vi "configuration UI.vi"() -> ()   [LabVIEW 2015, in "PID Module editor node.lvclass"]
uses:
  PID Module editor node.lvclass
  <vilib>/NI/Configuration Framework/Node/NodeRef.ctl
  <vilib>/NI/Configuration Framework/Node/NISE_CEF_Node.lvclass
  <vilib>/NI/AMC/Message Queue.ctl
  <vilib>/NI/AMC/Message.ctl
  <vilib>/NI/Tools/Keyed Array/KeyedArray.ctl
  <vilib>/NI/Configuration Framework/Node/UserEventRef.ctl
  <vilib>/NI/Configuration Framework/Controls/EventCluster.ctl
  <vilib>/NI/Configuration Framework/Node/StopEvent.ctl
  <vilib>/NI/Configuration Framework/Node/RefreshUIEvent.ctl
  <vilib>/NI/Configuration Framework/Node/CacheState.ctl
  <vilib>/NI/Configuration Framework/Node/NodeChangeEvent.ctl
  Program Files (x86)/National Instruments/LabVIEW 2013/vi.lib/NI/DCAF UI Toolkit/Controls/Configure.ctl
  <vilib>/NI/DCAF UI Toolkit/Controls/Remove.ctl
  <vilib>/NI/DCAF UI Toolkit/Controls/Add.ctl
  PID array element.ctl
  PID Module editor node.lvclass/PID Module editor node.ctl
  <vilib>/NI/Tag Bus Data Framework/Configuration Editor/Classes/Module editor node/module editor node.lvclass
  <vilib>/NI/Tag Bus Data Framework/Configuration Editor/Classes/Engine Parent/Engine Parent Editor Node.lvclass
  <vilib>/NI/Tools/Keyed Array/Tools_KeyedArray.lvlib
  <vilib>/NI/AMC/AMC.lvlib
  <vilib>/NI/Configuration Framework/NISE_CEF_TreeControl.lvlib
  module/configuration/PID Module configuration.lvclass
  <vilib>/NI/DCAF UI Toolkit/Controls/DCAF UI Elements.lvlib
panel:
  in  "node change":T1
  in  "cache state":T2
  in  "refresh UI":T3
  in  "stop event":T4
  in  "Tab Control":enum32{"Static Configuration"}(tab)
  in  "Down Button":bool
  in  "Up Button":bool
  in  "Last Button":bool
  in  "First Button":bool
  in  "Page Up Button":bool
  in  "Page Down Button":bool
  in  "Add Button":T5
  in  "Delete Button":T6
  in  "Settings Button":T7
  in  "hidden_remove":bool
  in  "hidden_settings":bool
  in  "hidden_Add":bool
  in  "PID Array":T8[](array[typedef])
  in  "user event":T9
  in  "main queue":T10
  in  "node ref":T11
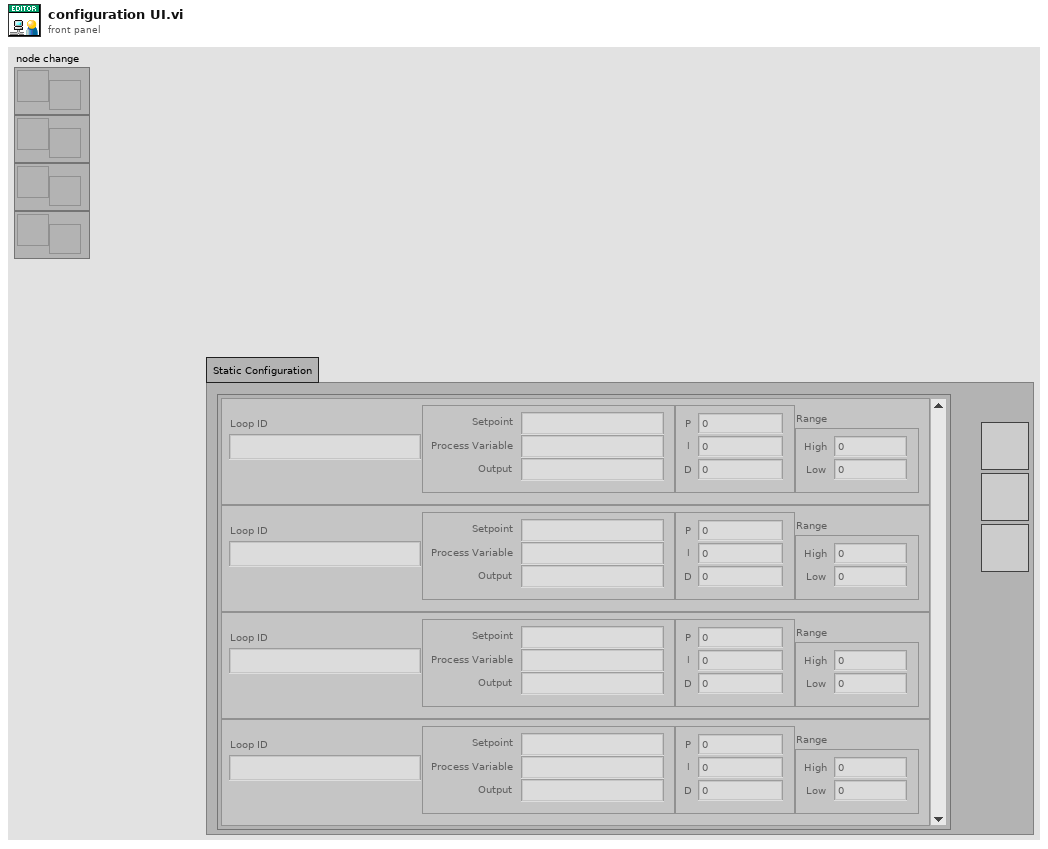
[diagram p1: front panel]
types:
  T1 = typedef "NISE_CEF_Node.lvclass/NodeChangeEvent.ctl" = refnum<user-event>
  T2 = typedef "NISE_CEF_Node.lvclass/CacheState.ctl" = refnum<user-event>
  T3 = typedef "NISE_CEF_Node.lvclass/RefreshUIEvent.ctl" = refnum<user-event>
  T4 = typedef "NISE_CEF_Node.lvclass/StopEvent.ctl" = refnum<user-event>
  T5 = typedef "DCAF UI Elements.lvlib/Add.ctl" = bool
  T6 = typedef "DCAF UI Elements.lvlib/Remove.ctl" = bool
  T7 = typedef "DCAF UI Elements.lvlib/Configure.ctl" = bool
  T8 = typedef "PID Module configuration.lvclass/PID array element.ctl" = cluster{"Loop ID":string, "Tags":cluster{"Setpoint":string, "Process Variable":string, "Output":string}, "Gains":cluster{"P":dbl, "I":dbl, "D":dbl}, "Range":cluster{"High":dbl, "Low":dbl}}
  T9 = typedef "NISE_CEF_Node.lvclass/UserEventRef.ctl" = refnum<user-event>
  T10 = typedef "AMC.lvlib/Message Queue.ctl" = refnum<queue>
  T11 = typedef "NISE_CEF_Node.lvclass/NodeRef.ctl" = refnum<data-value>
  T12 = enum8{"Enabled", "Disabled", "Disabled and Grayed Out"}
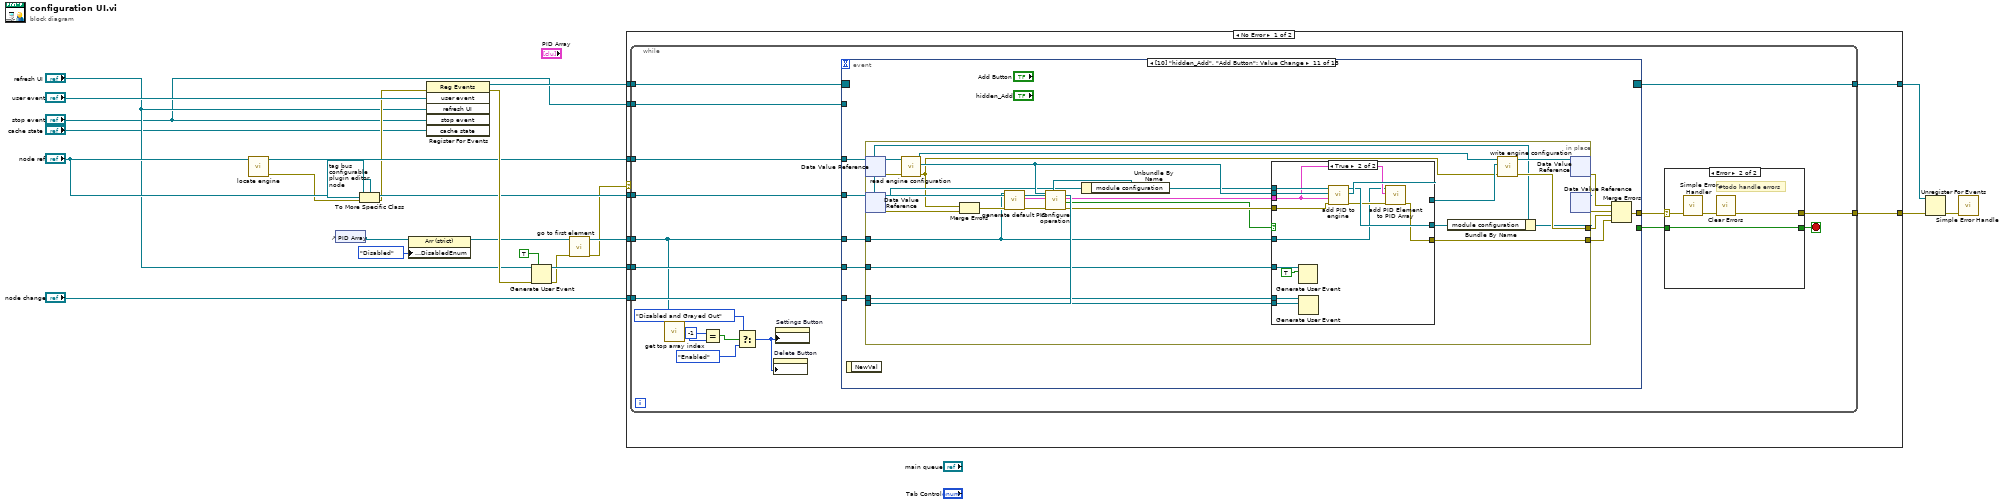
[diagram p0: block diagram]
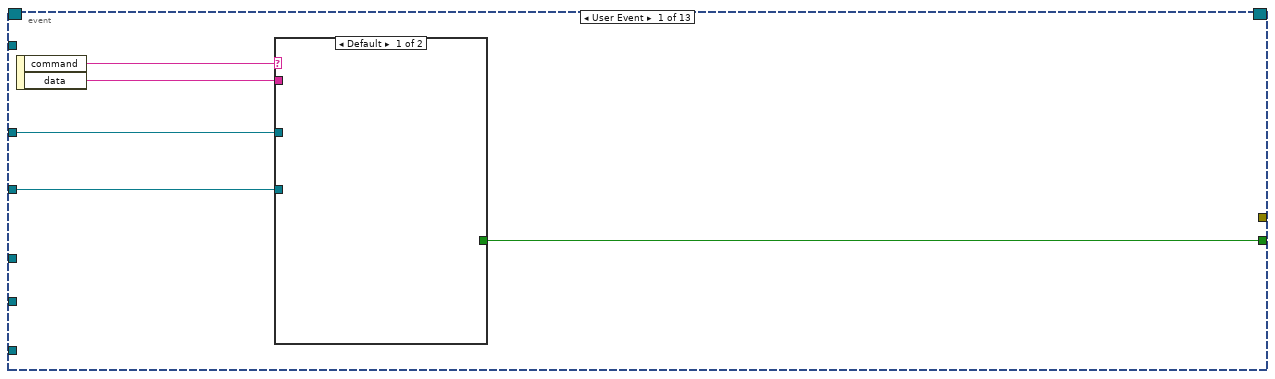
[diagram p2: hidden frame]
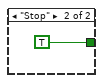
[diagram p3: hidden frame]
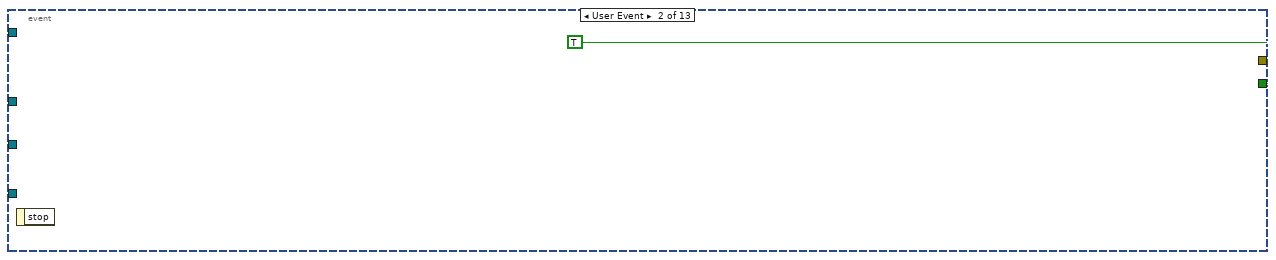
[diagram p4: hidden frame]
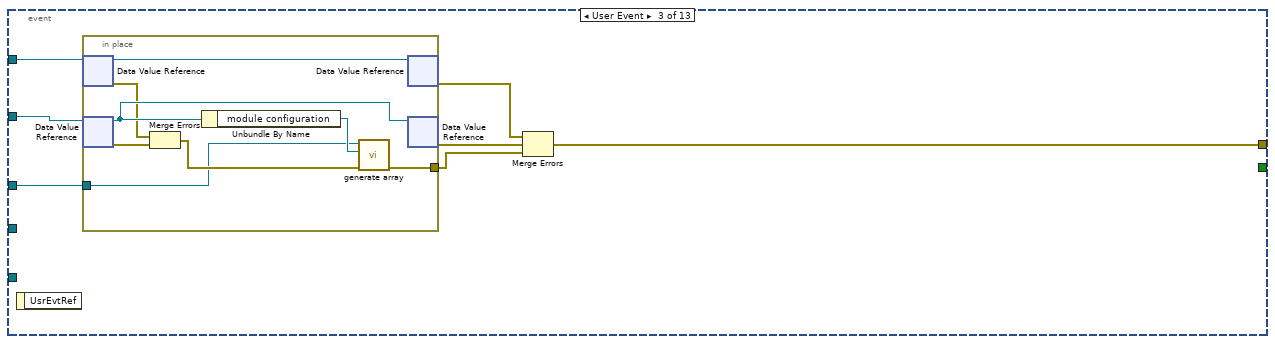
[diagram p5: hidden frame]
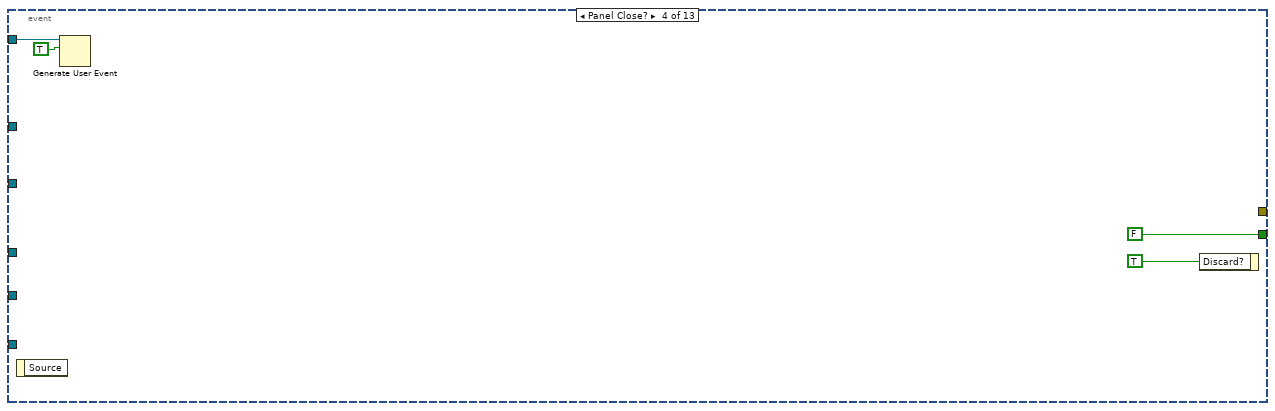
[diagram p6: hidden frame]
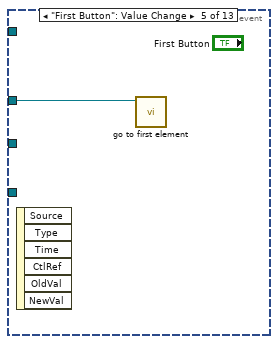
[diagram p7: hidden frame]
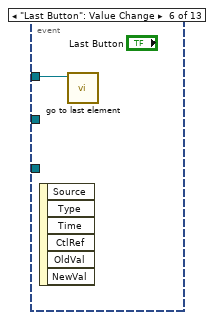
[diagram p8: hidden frame]
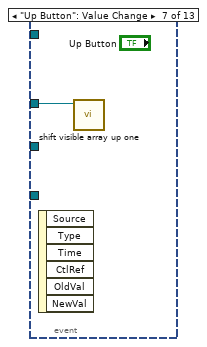
[diagram p9: hidden frame]
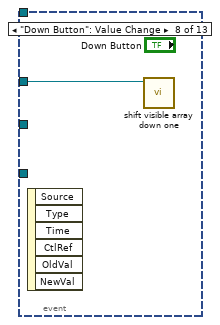
[diagram p10: hidden frame]
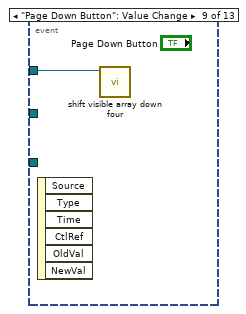
[diagram p11: hidden frame]
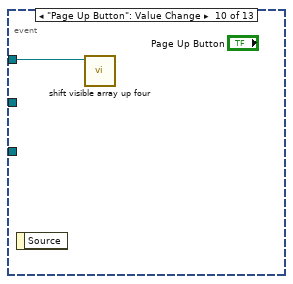
[diagram p12: hidden frame]
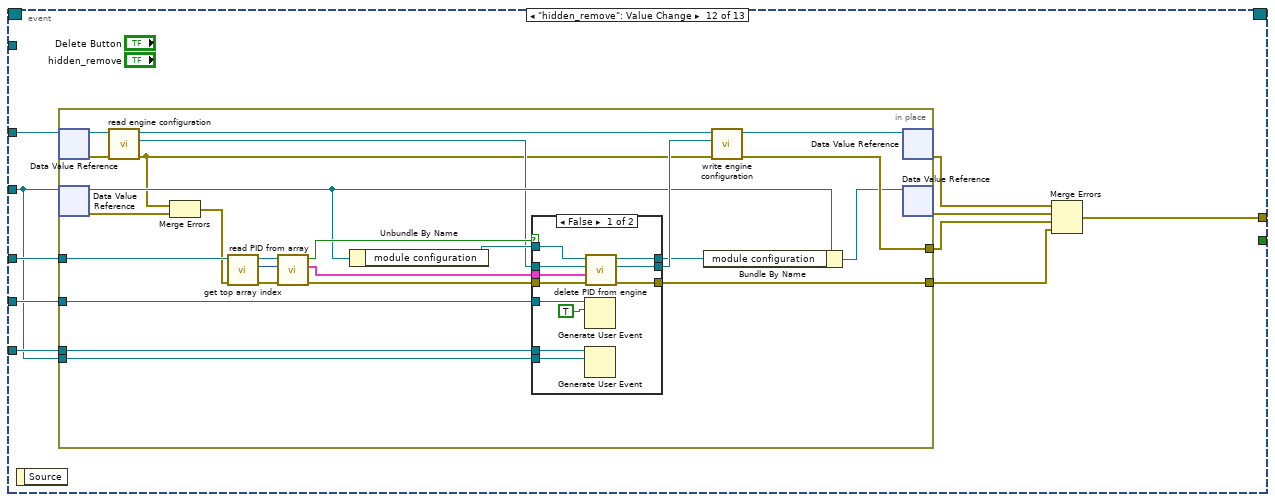
[diagram p14: hidden frame]
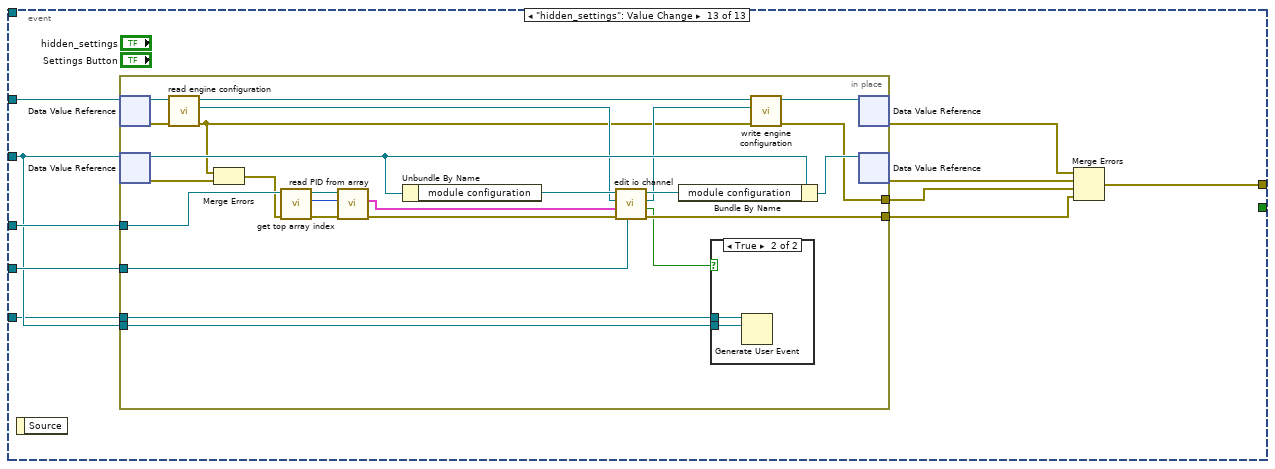
[diagram p16: hidden frame]
diagram:
  n1 = call <vilib>:"locate engine.vi"("component"="node ref") -> ("error out"=w13:errorcluster, "engine"=w19:refnum<data-value>)  [unwired: 9 in]
  n2 = control-ref of="PID Array"() -> (w1:refnum<vi>)
  n3 = To More Specific Class(target class=refnum<data-value> refnum ("data value reference"), reference="node ref", error in=w13) -> (specific class reference=w16:refnum<data-value>, error out=w15:errorcluster)
  n4 = property class="Arr (strict)"(reference=w1, "Array Element.DisabledEnum"=T12."Disabled" ("Disabled")) -> (reference out=w2:refnum<vi>)  [unwired: 1 in, 1 out]
  n5 = register-events(error in=w15, "user event", "refresh UI", "stop event", "cache state") -> (reference out=w24:refnum<event-registration>, error out=w20:errorcluster)  [unwired: 1 in]
  n6 = Generate User Event(user event="refresh UI", event data cluster=TRUE ("event data"), error in=w20) -> (user event out=w12:T3, error out=w5:errorcluster)  [unwired: 1 in]
  n7 = call "go to first element.vi"("error in (no error)"=w5, "Array in"=w2) -> ("error out"=w4:errorcluster, "Array out"=w6:refnum<vi>)  [unwired: 8 in]
  n8 = case shown="No Error" w4 {
    selector: w4 -> [_ w227]
    tunnel: w24 -> [w33 w226]
    tunnel: [w32 w226] -> w23
    tunnel: [w31 w227] -> w22
    tunnel: w19 -> [w30 _]
    tunnel: w6 -> [w29 _]
    tunnel: w16 -> [w28 _]
    tunnel: w12 -> [w27 _]
    tunnel: "node change" -> [w26 _]
    tunnel: "stop event" -> [w25 _]
    frame No Error {
      n9 = while {
        tunnel: w33 -> [w51]
        tunnel: [w50] -> w32
        tunnel: w28 -> [w47]
        tunnel: w30 -> [w46]
        tunnel: w27 -> [w45]
        tunnel: w29 -> [w37]
        tunnel: w26 -> [w44]
        tunnel: [w48] -> w31
        tunnel: w25 -> [w43]
        stop <- w49 stop-if-true
        n10 = call "get top array index.vi"("Array in"=w37) -> ("last value index"=w36:u32)  [unwired: 7 in, 3 out]
        n11 = Equal?(x=-1, y=w36) -> (x = y?=w34:bool)
        n12 = Select(t=T12."Disabled and Grayed Out", s=w34, f=T12."Enabled" ("Disabled")) -> (s? t:f=w38:T12)
        n13 = property on="Delete Button" class="Bool"("DisabledEnum"=w38) -> ()  [unwired: 2 in, 2 out]
        n14 = property on="Settings Button" class="Bool"("DisabledEnum"=w38) -> ()  [unwired: 2 in, 2 out]
        n15 = event shown="[10] \"hidden_Add\", \"Add Button\": Value Change" {
          selector: w51 -> [_ _ _ _ _ _ _ _ _ _ _ _ _]
          dyn-events: [_ _ _ _ _ _ _ _ _ _ _ _ _] -> w50
          timeout: _ -> [_ _ _ _ _ _ _ _ _ _ _ _ _]
          tunnel: [w56 TRUE _ FALSE _ _ _ _ _ _ _ _ _] -> w42
          tunnel: [_ _ w63 _ _ _ _ _ _ _ w84 w140 w190] -> w41
          tunnel: w47 -> [w54 _ w65 _ _ _ _ _ _ _ w90 w138 w188]
          tunnel: w46 -> [w53 _ w64 _ _ _ _ _ _ _ w91 w141 w189]
          tunnel: w45 -> [_ _ _ _ _ _ _ _ _ _ w93 w143 w192]
          tunnel: w37 -> [_ _ w59 _ w78 w79 w80 w81 w82 w83 w92 w142 w191]
          tunnel: w44 -> [_ _ _ _ _ _ _ _ _ _ w89 w139 w187]
          tunnel: w43 -> [_ _ _ w75 _ _ _ _ _ _ _ _ _]
          event User Event {
            n16 = event-data() -> ("command"=w55:string, "data"=w52:string)  [unwired: 1 in]
            n17 = case shown="Default" w55 {
              tunnel: [_ TRUE] -> w56
              tunnel: w54 -> [_ _]
              tunnel: w53 -> [_ _]
              tunnel: w52 -> [_ _]
              frame Default {
              }
              frame "Stop" {
              }
            }
          }
          event User Event {
            n18 = event-data() -> ()  [unwired: 1 in, 1 out]
          }
          event User Event {
            n19 = event-data() -> ()  [unwired: 1 in, 1 out]
            n20 = in-place {
              in-place-border: [w73] -> w60
              in-place-border: w59 -> [w66]
              n21 = in-place-dvr #1(w64) -> (w68:refnum<class "Engine Parent Editor Node.lvclass">, w69:errorcluster)
              n22 = in-place-dvr #2(w65) -> (w70:refnum<class "PID Module editor node.lvclass">, w71:errorcluster)
              n23 = Merge Errors(w69, w71) -> (w72:errorcluster)
              n24 = Unbundle By Name(w70) -> ("module configuration"=w67:refnum<class "PID Module configuration.lvclass">)
              n25 = call "generate array.vi"("error in"=w72, "tag bus configurable plugin module configuration"=w67, "array"=w66) -> ("error out"=w73:errorcluster)  [unwired: 8 in]
              n26 = in-place-dvr #1(w68) -> (w62:errorcluster)  [unwired: 1 out]
              n27 = in-place-dvr #2(w70) -> (w61:errorcluster)  [unwired: 1 out]
            }
            n28 = Merge Errors(w62, w61, w60) -> (w63:errorcluster)
          }
          event Panel Close? {
            n29 = event-data() -> ()  [unwired: 1 in, 1 out]
            n30 = Generate User Event(user event=w75, event data cluster=TRUE ("event data")) -> ()  [unwired: 2 in, 2 out]
            n31 = event-data("Discard?"=TRUE) -> ()  [unwired: 1 in, 1 out]
          }
          event "First Button": Value Change {
            n32 = event-data() -> ()  [unwired: 1 in, 6 out]
            n33 = call "go to first element.vi"("Array in"=w78) -> ()  [unwired: 9 in, 2 out]
          }
          event "Last Button": Value Change {
            n34 = event-data() -> ()  [unwired: 1 in, 6 out]
            n35 = call "go to last element.vi"("Array in"=w79) -> ()  [unwired: 9 in, 2 out]
          }
          event "Up Button": Value Change {
            n36 = event-data() -> ()  [unwired: 1 in, 6 out]
            n37 = call "shift visible array up one.vi"("Array in"=w80) -> ()  [unwired: 9 in, 2 out]
          }
          event "Down Button": Value Change {
            n38 = event-data() -> ()  [unwired: 1 in, 6 out]
            n39 = call "shift visible array down one.vi"("Array in"=w81) -> ()  [unwired: 9 in, 2 out]
          }
          event "Page Down Button": Value Change {
            n40 = event-data() -> ()  [unwired: 1 in, 6 out]
            n41 = call "shift visible array down four.vi"("Array in"=w82) -> ()  [unwired: 9 in, 2 out]
          }
          event "Page Up Button": Value Change {
            n42 = event-data() -> ()  [unwired: 1 in, 1 out]
            n43 = call "shift visible array up four.vi"("Array in"=w83) -> ()  [unwired: 9 in, 2 out]
          }
          event "hidden_Add": Value Change {
            n44 = event-data() -> ()  [unwired: 1 in, 1 out]
            n45 = in-place {
              in-place-border: [w96] -> w85
              in-place-border: w93 -> [w112]
              in-place-border: w92 -> [w97]
              in-place-border: [w108] -> w86
              in-place-border: w90 -> [w99]
              in-place-border: w89 -> [w98]
              n46 = in-place-dvr #3(w91) -> (w110:refnum<class "Engine Parent Editor Node.lvclass">, w95:errorcluster)
              n47 = in-place-dvr #4(w90) -> (w102:refnum<class "PID Module editor node.lvclass">, w103:errorcluster)
              n48 = call <vilib>:"read engine configuration.vi"("error in"=w95, "Engine Parent Editor Node in"=w110) -> ("error out"=w94:errorcluster, "engine configuration"=w105:refnum<class "engine configuration.lvclass">, "Engine Parent Editor Node out"=w107:refnum<class "Engine Parent Editor Node.lvclass">)  [unwired: 7 in]
              n49 = Merge Errors(w94, w103) -> (w111:errorcluster)
              n50 = call "generate default PID.vi"("error in"=w111, "PID array in"=w97) -> ("error out"=w116:errorcluster, "PID Array Element"=w117:T8)  [unwired: 8 in]
              n51 = Unbundle By Name(w102) -> ("module configuration"=w104:refnum<class "PID Module configuration.lvclass">)
              n52 = call "configure operation.vi"("tag bus configurable plugin module configuration"=w104, "error in"=w116, "line item in"=w117, "engine configuration"=w105) -> ("error out"=w114:errorcluster, "success"=w113:bool, "PID Loop out"=w115:T8)  [unwired: 4 in, 1 out]
              n53 = case shown="True" w113 {
                tunnel: [w120 w122] -> w96
                tunnel: w114 -> [w120 w125]
                tunnel: w105 -> [w119 w126]
                tunnel: w115 -> [_ w124]
                tunnel: w104 -> [w118 w127]
                tunnel: [w119 w133] -> w106
                tunnel: [w118 w132] -> w101
                tunnel: w112 -> [_ w131]
                tunnel: w99 -> [_ w129]
                tunnel: w98 -> [_ w128]
                tunnel: w97 -> [_ w121]
                frame False {
                }
                frame True {
                  n54 = Generate User Event(user event=w131, event data cluster=TRUE ("event data")) -> ()  [unwired: 2 in, 2 out]
                  n55 = Generate User Event(user event=w128, event data cluster=w129) -> ()  [unwired: 2 in, 2 out]
                  n56 = call "add PID to engine.vi"("error in (no error)"=w125, "PID element in"=w124, "engine configuration"=w126, "Tagbus PID Module configuration in"=w127) -> ("error out"=w123:errorcluster, "engine configuration out"=w133:refnum<class "engine configuration.lvclass">, "Tagbus PID Module configuration out"=w132:refnum<class "PID Module configuration.lvclass">)  [unwired: 5 in]
                  n57 = call "add PID Element to PID Array.vi"("error in"=w123, "PID Element"=w124, "PID Array ref in"=w121) -> ("error out"=w122:errorcluster)  [unwired: 8 in]
                }
              }
              n58 = Bundle By Name(cluster=w102, "module configuration"=w101) -> (w100:refnum<class "PID Module editor node.lvclass">)
              n59 = call <vilib>:"write engine configuration.vi"("error in"=w94, "engine configuration"=w106, "Engine Parent Editor Node in"=w107) -> ("error out"=w108:errorcluster, "Engine Parent Editor Node out"=w109:refnum<class "Engine Parent Editor Node.lvclass">)  [unwired: 7 in]
              n60 = in-place-dvr #3(w109) -> (w88:errorcluster)  [unwired: 1 out]
              n61 = in-place-dvr #4(w100) -> (w87:errorcluster)  [unwired: 1 out]
            }
            n62 = Merge Errors(w88, w87, w86, w85) -> (w84:errorcluster)
          }
          event "hidden_remove": Value Change {
            n63 = event-data() -> ()  [unwired: 1 in, 1 out]
            n64 = in-place {
              in-place-border: [w168] -> w134
              in-place-border: w143 -> [w164]
              in-place-border: w142 -> [w148]
              in-place-border: [w162] -> w135
              in-place-border: w139 -> [w151]
              in-place-border: w138 -> [w150]
              n65 = in-place-dvr #5(w141) -> (w159:refnum<class "Engine Parent Editor Node.lvclass">, w158:errorcluster)
              n66 = in-place-dvr #6(w138) -> (w157:refnum<class "PID Module editor node.lvclass">, w152:errorcluster)
              n67 = call <vilib>:"read engine configuration.vi"("error in"=w158, "Engine Parent Editor Node in"=w159) -> ("error out"=w153:errorcluster, "engine configuration"=w155:refnum<class "engine configuration.lvclass">, "Engine Parent Editor Node out"=w154:refnum<class "Engine Parent Editor Node.lvclass">)  [unwired: 7 in]
              n68 = Merge Errors(w153, w152) -> (w146:errorcluster)
              n69 = call "get top array index.vi"("error in (no error)"=w146, "Array in"=w148) -> ("error out"=w145:errorcluster, "top index"=w147:u32, "Array out"=w144:refnum<vi>)  [unwired: 6 in, 1 out]
              n70 = call "read PID from array.vi"("error in"=w145, "loop number"=w147, "PID Array"=w144) -> ("error out"=w165:errorcluster, "PID Array Element"=w166:T8, "empty tag?"=w167:bool)  [unwired: 6 in]
              n71 = Unbundle By Name(w157) -> ("module configuration"=w156:refnum<class "PID Module configuration.lvclass">)
              n72 = case shown="False" w167 {
                tunnel: [w174 w181] -> w168
                tunnel: w156 -> [w170 w180]
                tunnel: w155 -> [w169 w182]
                tunnel: w166 -> [w173 _]
                tunnel: w165 -> [w179 w181]
                tunnel: [w171 w182] -> w160
                tunnel: [w172 w180] -> w149
                tunnel: w164 -> [w178 _]
                tunnel: w151 -> [w177 _]
                tunnel: w150 -> [w176 _]
                frame False {
                  n73 = Generate User Event(user event=w178, event data cluster=TRUE ("event data")) -> ()  [unwired: 2 in, 2 out]
                  n74 = Generate User Event(user event=w177, event data cluster=w176) -> ()  [unwired: 2 in, 2 out]
                  n75 = call "delete PID from engine.vi"("error in (no error)"=w179, "PID Loop in"=w173, "engine configuration in"=w169, "Tagbus PID Module configuration in"=w170) -> ("error out"=w174:errorcluster, "engine configuration out"=w171:refnum<class "engine configuration.lvclass">, "Tagbus PID Module configuration out"=w172:refnum<class "PID Module configuration.lvclass">)  [unwired: 4 in, 1 out]
                }
                frame True {
                }
              }
              n76 = Bundle By Name(cluster=w157, "module configuration"=w149) -> (w161:refnum<class "PID Module editor node.lvclass">)
              n77 = call <vilib>:"write engine configuration.vi"("error in"=w153, "engine configuration"=w160, "Engine Parent Editor Node in"=w154) -> ("error out"=w162:errorcluster, "Engine Parent Editor Node out"=w163:refnum<class "Engine Parent Editor Node.lvclass">)  [unwired: 7 in]
              n78 = in-place-dvr #5(w163) -> (w137:errorcluster)  [unwired: 1 out]
              n79 = in-place-dvr #6(w161) -> (w136:errorcluster)  [unwired: 1 out]
            }
            n80 = Merge Errors(w137, w136, w135, w134) -> (w140:errorcluster)
          }
          event "hidden_settings": Value Change {
            n81 = event-data() -> ()  [unwired: 1 in, 1 out]
            n82 = in-place {
              in-place-border: [w217] -> w183
              in-place-border: w192 -> [w216]
              in-place-border: w191 -> [w200]
              in-place-border: [w209] -> w184
              in-place-border: w188 -> [w203]
              in-place-border: w187 -> [w202]
              n83 = in-place-dvr #7(w189) -> (w212:refnum<class "Engine Parent Editor Node.lvclass">, w211:errorcluster)
              n84 = in-place-dvr #8(w188) -> (w215:refnum<class "PID Module editor node.lvclass">, w197:errorcluster)
              n85 = call <vilib>:"read engine configuration.vi"("error in"=w211, "Engine Parent Editor Node in"=w212) -> ("error out"=w196:errorcluster, "engine configuration"=w205:refnum<class "engine configuration.lvclass">, "Engine Parent Editor Node out"=w207:refnum<class "Engine Parent Editor Node.lvclass">)  [unwired: 7 in]
              n86 = Merge Errors(w196, w197) -> (w195:errorcluster)
              n87 = call "get top array index.vi"("error in (no error)"=w195, "Array in"=w200) -> ("error out"=w198:errorcluster, "top index"=w199:u32, "Array out"=w193:refnum<vi>)  [unwired: 6 in, 1 out]
              n88 = call "read PID from array.vi"("error in"=w198, "loop number"=w199, "PID Array"=w193) -> ("error out"=w194:errorcluster, "PID Array Element"=w201:T8)  [unwired: 6 in, 1 out]
              n89 = Unbundle By Name(w215) -> ("module configuration"=w208:refnum<class "PID Module configuration.lvclass">)
              n90 = call "edit io channel.vi"("refresh UI"=w216, "error in"=w194, "PID Loop Element"=w201, "engine configuration in"=w205, "tag bus configurable plugin module configuration in"=w208) -> ("error out"=w217:errorcluster, "change?"=w204:bool, "engine configuration"=w206:refnum<class "engine configuration.lvclass">, "tag bus configurable plugin module configuration out"=w213:refnum<class "PID Module configuration.lvclass">)  [unwired: 3 in]
              n91 = Bundle By Name(cluster=w215, "module configuration"=w213) -> (w214:refnum<class "PID Module editor node.lvclass">)
              n92 = case shown="True" w204 {
                tunnel: w203 -> [_ w219]
                tunnel: w202 -> [_ w218]
                frame False {
                }
                frame True {
                  n93 = Generate User Event(user event=w218, event data cluster=w219) -> ()  [unwired: 2 in, 2 out]
                }
              }
              n94 = call <vilib>:"write engine configuration.vi"("error in"=w196, "engine configuration"=w206, "Engine Parent Editor Node in"=w207) -> ("error out"=w209:errorcluster, "Engine Parent Editor Node out"=w210:refnum<class "Engine Parent Editor Node.lvclass">)  [unwired: 7 in]
              n95 = in-place-dvr #7(w210) -> (w186:errorcluster)  [unwired: 1 out]
              n96 = in-place-dvr #8(w214) -> (w185:errorcluster)  [unwired: 1 out]
            }
            n97 = Merge Errors(w186, w185, w184, w183) -> (w190:errorcluster)
          }
        }
        n98 = case shown="Error" w41 {
          selector: w41 -> [w220 w224]
          tunnel: [w221 w225] -> w49
          tunnel: w42 -> [w221 w225]
          tunnel: [w220 w222] -> w48
          frame No Error {
          }
          frame Error {
            # "#todo handle errors"
            n99 = call <vilib>:"Simple Error Handler.vi"("error in (no error)"=w224) -> ("error out"=w223:errorcluster)  [unwired: 4 in, 4 out]
            n100 = call <vilib>:"Clear Errors.vi"("error in (no error)"=w223) -> ("error out"=w222:errorcluster)  [unwired: 5 in, 1 out]
          }
        }
      }
    }
    frame Error {
    }
  }
  n101 = Unregister For Events(event registration refnum=w23, error in=w22) -> (error out=w18:errorcluster)
  n102 = call <vilib>:"Simple Error Handler.vi"("error in (no error)"=w18) -> ()  [unwired: 4 in, 5 out]
